vi "SessionBank.vi"(7 "Action (Get)":T1=enum."Get", 8 "error in (no error)":errorcluster, 11 "PythonSession in":refnum<class "PythonSession.lvclass">) -> (0 "error out":errorcluster, 3 "PythonSession out":refnum<class "PythonSession.lvclass">)   [LabVIEW 2022 SP3, in "PythonWrapper.lvlib" / "PythonSession.lvclass"]
uses:
  PythonSession.lvclass
  _BankAction.ctl
  PythonSession.lvclass/PythonSession.ctl
  _BankData.ctl
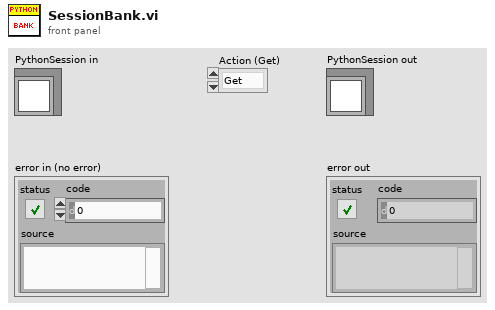
[diagram p1: front panel]
types:
  T1 = typedef "PythonWrapper.lvlib/PythonSession.lvclass/_BankAction.ctl" = enum16{"Add", "Get", "Remove"}
  T2 = typedef "PythonWrapper.lvlib/PythonSession.lvclass/_BankData.ctl" = cluster{"PythonSession":refnum<k35>, "ReferenceCounter":u32}
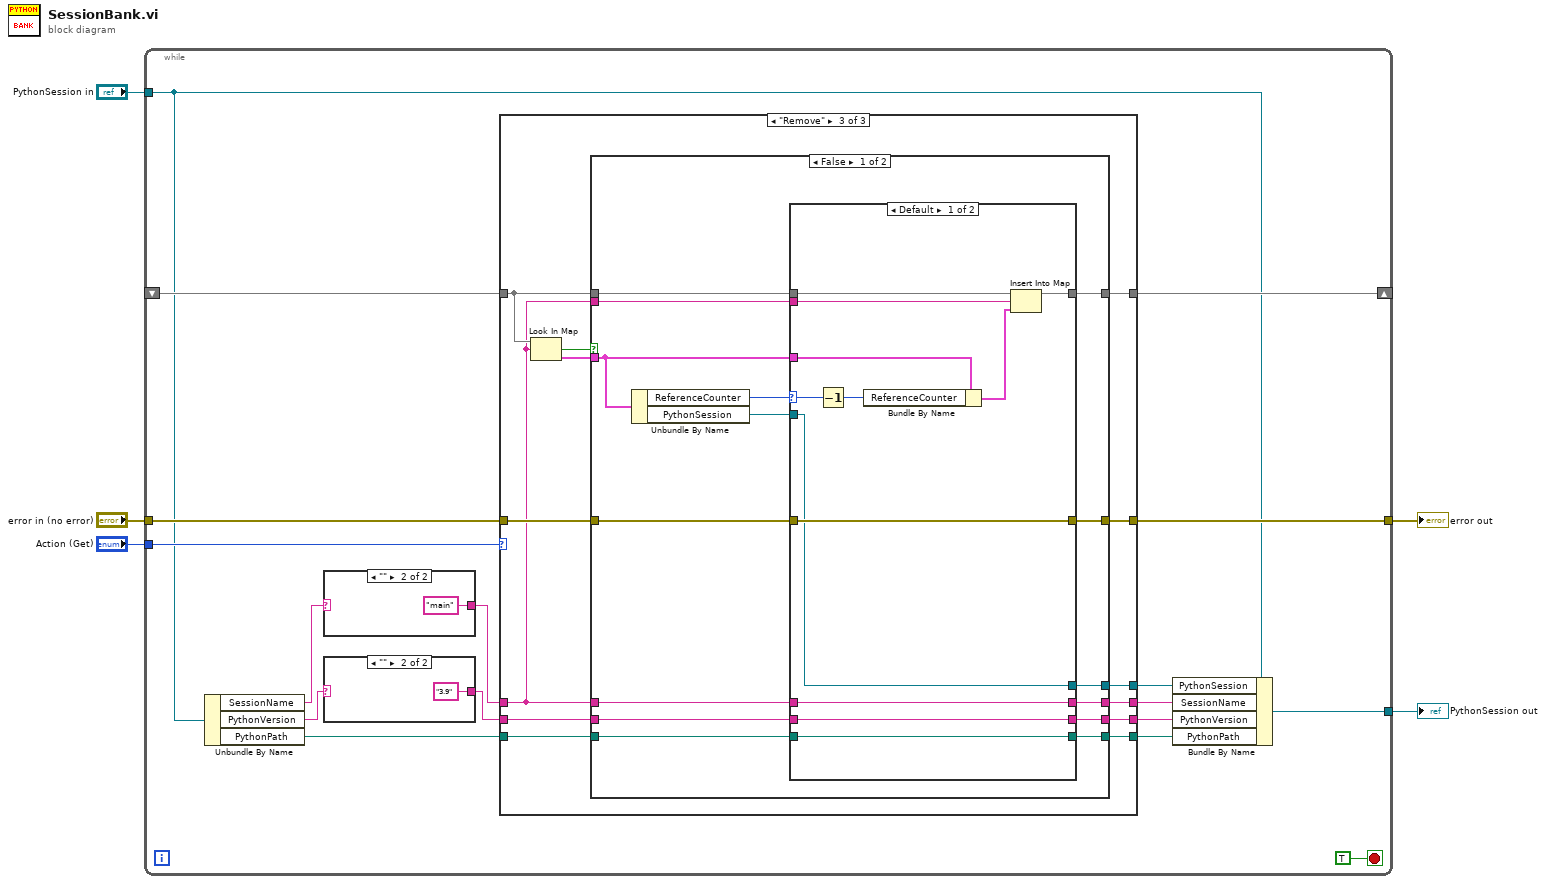
[diagram p0: block diagram]
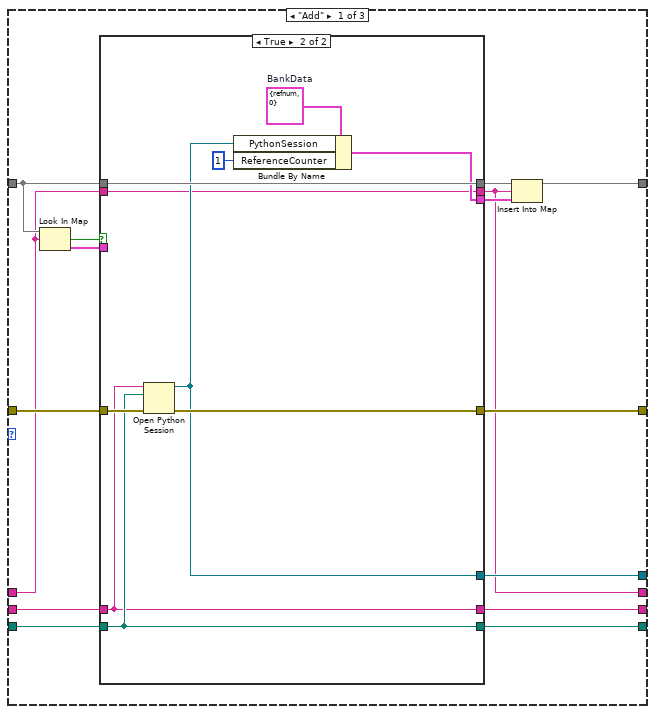
[diagram p4: hidden frame]
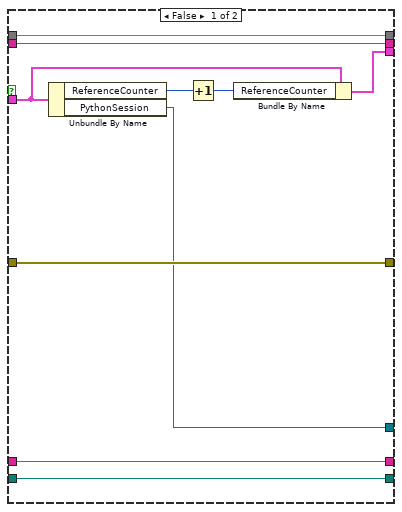
[diagram p5: hidden frame]
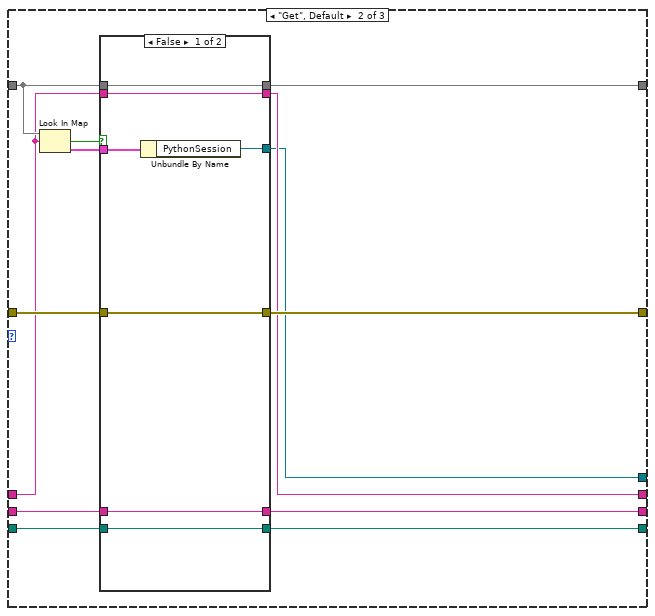
[diagram p6: hidden frame]
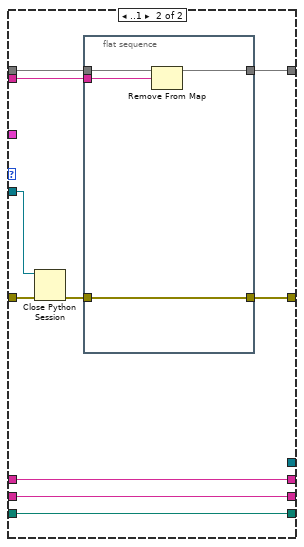
[diagram p8: hidden frame]
diagram:
  n1 = while {
    tunnel: "Action (Get)" -> [w21]
    shift-right: [w17] -> _
    shift-left: _ -> [w20]
    tunnel: "PythonSession in" -> [w15]
    tunnel: "error in (no error)" -> [w19]
    tunnel: [w18] -> w2
    tunnel: [w10] -> w1
    stop <- TRUE stop-if-true
    n2 = Unbundle By Name(w15) -> ("SessionName"=w14:string, "PythonVersion"=w13:string, "PythonPath"=w16:path)
    n3 = case shown="\"\"" w14 {
      selector: w14 -> [w25 _]
      tunnel: [w25 "main"] -> w7
      frame Default {
      }
      frame "" {
      }
    }
    n4 = case shown="\"\"" w13 {
      selector: w13 -> [w23 _]
      tunnel: [w23 "3.9"] -> w9
      frame Default {
      }
      frame "" {
      }
    }
    n5 = case shown="\"Remove\"" w21 {
      tunnel: w20 -> [w40 w73 w95]
      tunnel: w19 -> [w39 w72 w99]
      tunnel: [w38 w71 w97] -> w18
      tunnel: w9 -> [w37 w70 w90]
      tunnel: w16 -> [w36 w69 w92]
      tunnel: [w33 w67 w98] -> w17
      tunnel: [w28 w66 w89] -> w8
      tunnel: [w29 w65 w88] -> w6
      tunnel: [w30 w64 w91] -> w12
      tunnel: [w31 w63 w93] -> w11
      tunnel: w7 -> [w27 w62 w87]
      frame "Add" {
        n6 = Look In Map(map=w40, key=w27) -> (key not found?=w41:bool, value=w35:T2)  [unwired: 1 in]
        n7 = case shown="True" w41 {
          tunnel: w40 -> [w47 w61]
          tunnel: w27 -> [w46 w52]
          tunnel: w39 -> [w51 w60]
          tunnel: [w51 w59] -> w38
          tunnel: w37 -> [w49 w57]
          tunnel: w36 -> [w50 w58]
          tunnel: [w47 w61] -> w34
          tunnel: w35 -> [w45 _]
          tunnel: [w48 w55] -> w29
          tunnel: [w50 w58] -> w31
          tunnel: [w49 w57] -> w30
          tunnel: [w46 w52] -> w28
          tunnel: [w43 w54] -> w32
          frame False {
            n8 = Unbundle By Name(w45) -> ("ReferenceCounter"=w42:u32, "PythonSession"=w48:refnum<k35>)
            n9 = Increment(x=w42) -> (x+1=w44:u32)
            n10 = Bundle By Name(cluster=w45, "ReferenceCounter"=w44) -> (w43:T2)
          }
          frame True {
            w56 = T2 {"PythonSession"=refnum, "ReferenceCounter"=0}  # BankData
            n11 = Open Python Session(python version=w57, python path=w58, 3:w60) -> (session out=w55:refnum<k35>, error out=w59:errorcluster)
            n12 = Bundle By Name(cluster=w56, "PythonSession"=w55, "ReferenceCounter"=u32 1) -> (w54:T2)
          }
        }
        n13 = Insert Into Map(map in=w34, key=w28, value=w32) -> (map out=w33:map{string, T2})  [unwired: 2 out]
      }
      frame "Get", Default {
        n14 = Look In Map(map=w73, key=w62) -> (key not found?=w74:bool, value=w68:T2)  [unwired: 1 in]
        n15 = case shown="False" w74 {
          tunnel: w73 -> [w76 w86]
          tunnel: w62 -> [w75 w84]
          tunnel: w72 -> [w81 w85]
          tunnel: [w81 w85] -> w71
          tunnel: w70 -> [w79 w83]
          tunnel: w69 -> [w80 w82]
          tunnel: [w76 w86] -> w67
          tunnel: w68 -> [w77 _]
          tunnel: [w78 _] -> w65
          tunnel: [w80 w82] -> w63
          tunnel: [w79 w83] -> w64
          tunnel: [w75 w84] -> w66
          frame False {
            n16 = Unbundle By Name(w77) -> ("PythonSession"=w78:refnum<k35>)
          }
          frame True {
          }
        }
      }
      frame "Remove" {
        n17 = Look In Map(map=w95, key=w87) -> (key not found?=w94:bool, value=w96:T2)  [unwired: 1 in]
        n18 = case shown="False" w94 {
          tunnel: w99 -> [w114 w144]
          tunnel: [w113 w145] -> w98
          tunnel: [w112 w144] -> w97
          tunnel: w96 -> [w108 _]
          tunnel: w95 -> [w111 w145]
          tunnel: w87 -> [w110 _]
          tunnel: [w107 w143] -> w93
          tunnel: w92 -> [w106 w143]
          tunnel: w90 -> [w104 w142]
          tunnel: [w105 w142] -> w91
          tunnel: w87 -> [w103 w141]
          tunnel: [w102 w141] -> w89
          tunnel: [w101 _] -> w88
          frame False {
            n19 = Unbundle By Name(w108) -> ("ReferenceCounter"=w109:u32, "PythonSession"=w100:refnum<k35>)
            n20 = case shown="Default" w109 {
              selector: w109 -> [w122 _]
              tunnel: w114 -> [w125 w136]
              tunnel: [w125 w134] -> w112
              tunnel: w111 -> [w126 w133]
              tunnel: [w124 w132] -> w113
              tunnel: w110 -> [w123 w131]
              tunnel: w108 -> [w119 _]
              tunnel: [w118 w130] -> w107
              tunnel: w106 -> [w118 w130]
              tunnel: [w117 w129] -> w105
              tunnel: w104 -> [w117 w129]
              tunnel: w103 -> [w116 w128]
              tunnel: [w116 w128] -> w102
              tunnel: w100 -> [w115 w127]
              tunnel: [w115 _] -> w101
              frame Default {
                n21 = Decrement(x=w122) -> (x-1=w121:u32)
                n22 = Bundle By Name(cluster=w119, "ReferenceCounter"=w121) -> (w120:T2)
                n23 = Insert Into Map(map in=w126, key=w123, value=w120) -> (map out=w124:map{string, T2})  [unwired: 2 out]
              }
              frame ..1 {
                n24 = Close Python Session(session in=w127, error in=w136) -> (11:w135:errorcluster)
                n25 = flat-sequence {
                  tunnel: w135 -> [w137]
                  tunnel: [w137] -> w134
                  tunnel: w133 -> [w140]
                  tunnel: [w139] -> w132
                  tunnel: w131 -> [w138]
                  frame #0 {
                    n26 = Remove From Map(10:w138, 11:w140) -> (3:w139:map{string, T2})  [unwired: 2 out]
                  }
                }
              }
            }
          }
          frame True {
          }
        }
      }
    }
    n27 = Bundle By Name(cluster=w15, "PythonSession"=w6, "SessionName"=w8, "PythonVersion"=w12, "PythonPath"=w11) -> (w10:refnum<class "PythonSession.lvclass">)
  }
  "PythonSession out" <- w1
  "error out" <- w2
